vi "NewROI.vi"(11 "MagAnalysis_Online in":refnum<class "MagAnalysis_Online.lvclass">) -> (3 "MagAnalysis_Online out":refnum<class "MagAnalysis_Online.lvclass">)   [LabVIEW 2020, in "MagAnalysis_Online.lvclass"]
uses:
  MagAnalysis_Online.lvclass
  specClustercommandTypdef.ctl
  MagAnalysis_Online.lvclass/MagAnalysis_Online.ctl
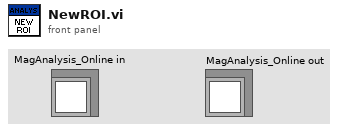
[diagram p1: front panel]
types:
  T1 = typedef "specClustercommandTypdef.ctl" = enum16{"init", "addCluster", "read", "clear"}
  T2 = typedef "MagAnalysis_Online.lvclass/settings_TypDef.ctl" = cluster{"CamSettings":T3, "timeout":T8, "Screws":T10, "number of cam":dbl, "X size":dbl, "srewstart":T13, "Save":T6, "offset":dbl, "localsavingpath":path, "ROIString":string, "exposure":T8, "trigger":T6}
  T3 = typedef "CamSettings_Typdef.ctl" = cluster{"Cam 0":T4, "Cam 1":T4, "Cam 2":T4, "Cam 3":T4}
  T4 = typedef "CamSettingSUB_TypDEf.ctl" = cluster{"position":dbl, "pixelsize":dbl, "start":dbl, "end":dbl, "center":dbl, "Lens":T5, "Forward":T6, "Spec_Calib_file 2":path, "map":path, "y size":i32, "UserROI":T7, "CamMaxPixel":cluster{"X":i32, "Y":i32}, "CamROI":T9}
  T5 = typedef "CamAndObj_TypDEf.ctl" = enum16{"FL1-f8x08", "FL1-f8x06", "FL1-f8", "ch300-f50", "FL2G-f8", "FL3M14-f8", "FL3M14-f8x08", "FL3M14-f8x08(2x2)"}
  T6 = typedef "OnOffTypeDef.ctl" = enum16{"off", "on"}
  T7 = typedef "userROI.ctl" = cluster{"Width":T8, "Hight":T8, "OffsetX":T8, "OffsetY":T8}
  T8 = typedef "BaseDriver.lvclass/numericVariable_TypeDef.ctl" = cluster{"Value":dbl, "Min":dbl, "Max":dbl, "StepSize":dbl, "Tolerance":dbl, "ValueActual":dbl}
  T9 = typedef "CamRoiTypDef.ctl" = cluster{"Width":dbl, "Hight":dbl, "OffsetX":dbl, "OffsetY":dbl}
  T10 = typedef "SrewMaster_TYpDef.ctl" = cluster{"Cam 0":T11, "Cam 1":T11, "Cam 2":T11, "Cam 3":T11}
  T11 = typedef "srew_TypDEf.ctl" = cluster{"S 0":T12, "S 1":T12, "S 2":T12, "S 3":T12, "S 4":T12, "S 5":T12}
  T12 = typedef "ScrewSub_Typdef.ctl" = cluster{"0":i32, "1":i32, "2":i32, "3":i32}
  T13 = typedef "screwstart.ctl" = cluster{"Cam 0":dbl, "Cam 1":dbl, "Cam 2":dbl, "Cam 3":dbl}
  T14 = typedef "fileCalib.ctl" = cluster{"Cam 1":T15, "Cam 2":T15, "Cam 3":T15, "Cam 4":T15}
  T15 = typedef "configTypDEf.ctl" = cluster{"bending angle":dbl[], "screen [m]":dbl[], "momentum [MeV/c]":dbl[], "total path [m]":dbl[], "x[mm](rms)":dbl[], "x[mm](rms,b)":dbl[], "y[mm](rms)":dbl[], "y[mm](rms,b)":dbl[]}
  T16 = typedef "calib_Sub_Typdef.ctl" = cluster{"incident ANGLE COMPENSATION":dbl[], "dp/B [MeV/C/B]":dbl[], "charge compensation":dbl[], "Momentum [MeV/C]":dbl[], "energyDependence Input":dbl[], "pixel angle (y)":dbl[], "dp [MeV/C/] ":dbl[], "angle 2Dfor spectrumj":dbl[][], "dp [MeV/C] 2D":dbl[][], "charge compensation 2D":dbl[][], "Screen&Camera 2":T17, "ROI info":T18, "Y 2D full angle":dbl[][], "calib pixel":T19, "2D":T20, "UserROI":T9, "final":T21, "B[T]":dbl, "index":dbl}
  T17 = typedef "ScreenCam2_TypDEf.ctl" = cluster{"Screen Orientation":string, "Screen angle":string, "Lens":T5, "Calibration (mm/pix)":dbl}
  T18 = typedef "ROIInfo_TypDef.ctl" = cluster{"npix-X":i32, "npix-Y":i32, "Left [pix]":dbl, "Top [pix]":dbl}
  T19 = typedef "calibPixel.ctl" = cluster{"y1(pixel)":dbl[], "y2(pixel)":dbl[], "dp/B [MeV/C/B] (pixel)":dbl[], "energyDependence Input(pixel)":dbl[], "bending angle [deg](pixel)":dbl[], "total path(pixel)":dbl[], "pixel angle (y)(pixel)":dbl[], "energy dependence (pixel)":dbl[], "charge compensation (pixel)":dbl[], "Momentum [MeV/C](pixel)":dbl[], "angular compensation(pixel)":dbl[]}
  T20 = typedef "2DTypDef.ctl" = cluster{"dp":dbl[][], "chargeCompensation":dbl[][], "angle":dbl[][], "Momentum":dbl[][]}
  T21 = typedef "finalCalibTypdef.ctl" = cluster{"X":dbl[][], "xi":dbl[][], "delta momentum":dbl, "Y":dbl[][], "yi":dbl[][], "angle (Y)":dbl[], "delta angle":dbl, "scale delta angle":dbl, "intraX":dbl, "intraY":dbl, "mask":dbl[][]}
  T22 = cluster{"[0]":T16, "[1]":T16, "[2]":T16, "[3]":T16}
  T23 = cluster{"[0]":T15, "[1]":T15, "[2]":T15, "[3]":T15}
  T24 = typedef "Calib_Typdef.ctl" = cluster{"cam 0":T16, "cam 1":T16, "cam 2":T16, "cam 3":T16}
  T25 = cluster{"S 0":i32[][], "S 1":i32[][], "S 2":i32[][], "S 3":i32[][]}
  T26 = typedef "reshapeINfo_TypDef.ctl" = cluster{"emptyImageArray":dbl[], "max Y size":i32, "X size":i32, "number of cam":i32, "emptyZArrayforreshape":T27}
  T27 = typedef "emptyArray_TYpDEf.ctl" = cluster{"Cam 0":T28, "Cam 1":T28, "Cam 2":T28, "Cam 3":T28}
  T28 = typedef "emptyArrayCamX_TypDef.ctl" = cluster{"1":dbl[][], "2":dbl[][]}
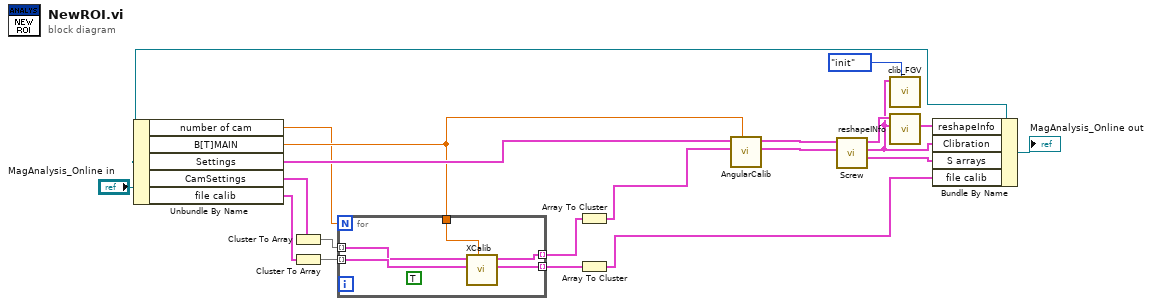
[diagram p0: block diagram]
diagram:
  n1 = Unbundle By Name("MagAnalysis_Online in") -> ("number of cam"=w1:dbl, "B[T]MAIN"=w2:dbl, "Settings"=w17:T2, "CamSettings"=w7:T3, "file calib"=w8:T14)
  n2 = Cluster To Array(cluster=w7) -> (array=w6:T4[])
  n3 = Cluster To Array(cluster=w8) -> (array=w9:T15[])
  n4 = for {
    N: w1 -> [_]
    tunnel: [w25] -> w10 mode=indexing
    tunnel: [w24] -> w11 mode=indexing
    tunnel: w9 -> [w23] mode=indexing
    tunnel: w6 -> [w22] mode=indexing
    tunnel: w2 -> [w21]
    (unwired) TRUE ("New (one file)")
    n5 = call "XCalib.vi"("B [T]"=w21, "fileCalib"=w23, "DB calib"=w22) -> ("fileCalib out"=w24:T15, "cam calib"=w25:T16)  [unwired: 6 in, 1 out]
  }
  n6 = Array To Cluster(array=w10) -> (cluster=w4:T22)
  n7 = Array To Cluster(array=w11) -> (cluster=w5:T23)
  n8 = call "AngularCalib.vi"("B [T]"=w2, "Clibration"=w4, "Settings"=w17) -> ("Clibration 2"=w3:T24, "Settings OUT"=w16:T2)  [unwired: 7 in]
  n9 = call "Screw.vi"("Clibration 2"=w3, "Settings in"=w16) -> ("S arrays"=w15:T25, "Clibration 2"=w12:T24, "Settings out"=w14:T2)  [unwired: 7 in]
  n10 = call "clib_FGV.vi"("command"=specClustercommandTypdef."init", "Clibration"=w12) -> ()  [unwired: 8 in, 2 out]
  n11 = call "reshapeINfo.vi"("Clibration"=w12, "Settings"=w14) -> ("reshapeInfo out"=w18:T26)  [unwired: 9 in]
  n12 = Bundle By Name(cluster="MagAnalysis_Online in", "reshapeInfo"=w18, "Clibration"=w12, "S arrays"=w15, "file calib"=w5) -> (→"MagAnalysis_Online out":refnum<class "MagAnalysis_Online.lvclass">)
